vi "winFormsSubVI searchLayout.vi"(8 "error in (no error)":errorcluster, 11 "searchString":refnum<vi>) -> (0 "error out":errorcluster)   [LabVIEW 2018]
uses:
  PublicSubVI/Class/QMH/QMH.lvclass
panel:
  in  "cancelBtn":bool
  in  "searchBtn":bool
  in  "searchText":string caption="Search Text :"
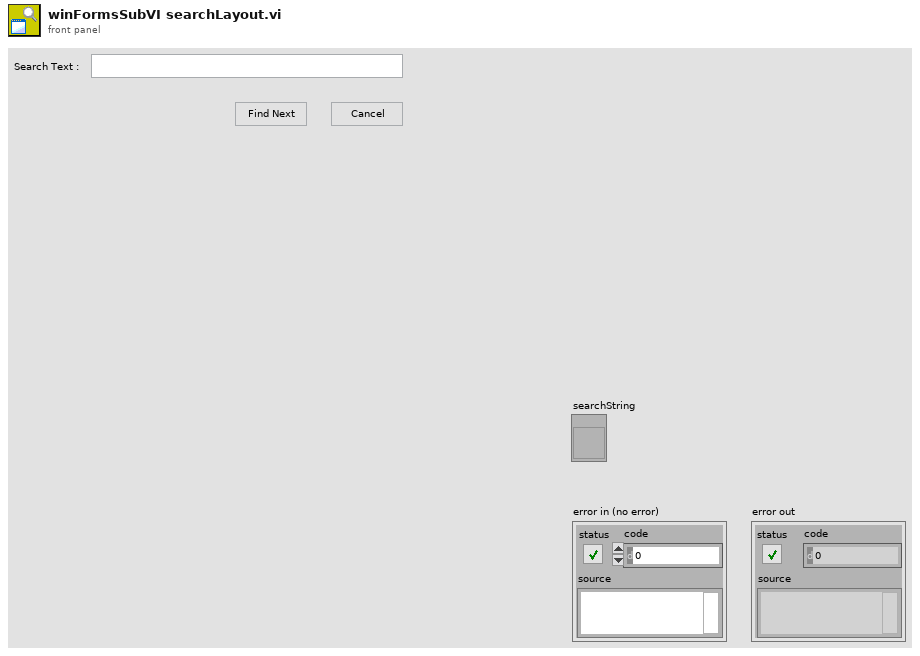
[diagram p1: front panel]
types:
  T1 = enum32{"Invalid", "Default", "Floating", "Floating/Auto-Hide", "Modal"}
  T2 = typedef "eventvkey.ctl" = enum16{"ASCII", "Enter", "Return", "Shift", "Ctrl", "Alt", "Cmd", "Opt", "Caps", "NumLock", "Clear", "Break", "Up", "Down", "Left", "Right", "Insert", "Delete", "Home", "End", "PageUp", "PageDown", "Escape", "Help", "Pause", "ScrollLock", "F1", "F2", "F3", "F4", "F5", "F6", "F7", "F8", "F9", "F10", "F11", "F12", "F13", "F14", "F15", "F16", "F17", "F18", "F19", "F20", "F21", "F22", "F23", "F24", "Play", "VolumeUp", "VolumeDown", "Mute", "Two Byte Char"}
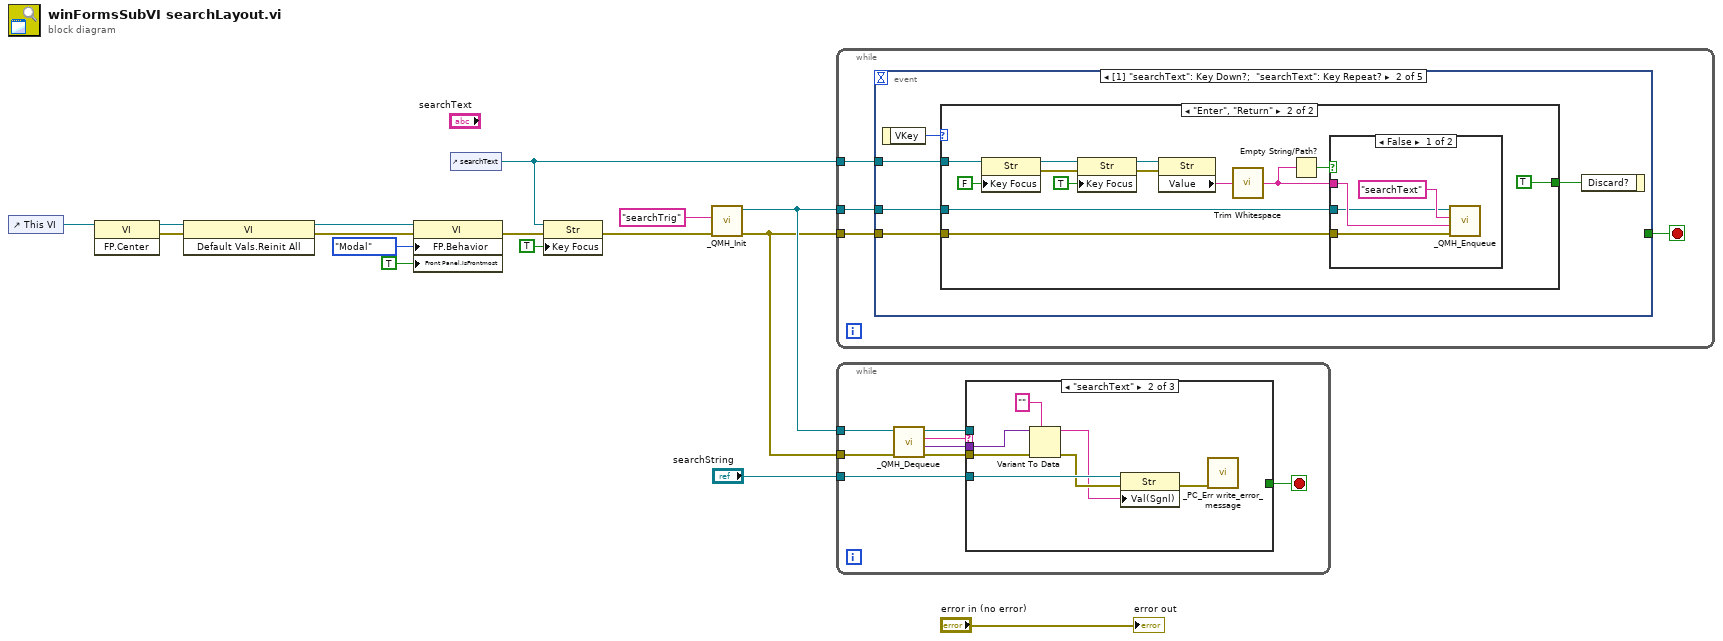
[diagram p0: block diagram]
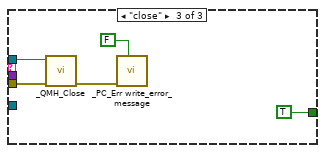
[diagram p3: hidden frame]
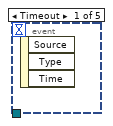
[diagram p4: hidden frame]
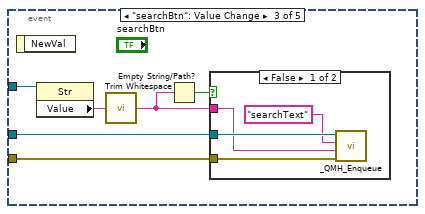
[diagram p7: hidden frame]
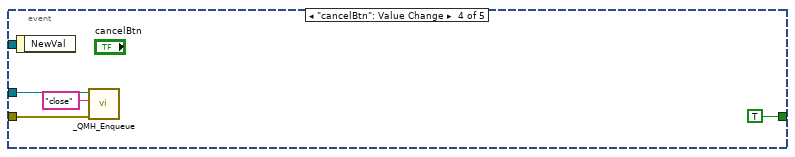
[diagram p9: hidden frame]
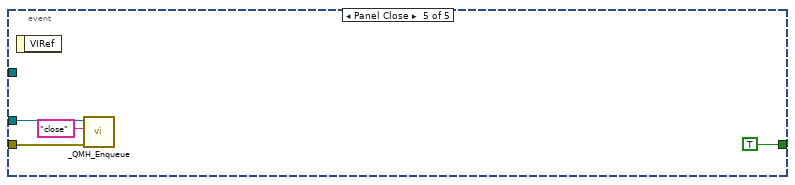
[diagram p10: hidden frame]
diagram:
  n1 = control-ref of="This VI"() -> (w9:refnum<vi>)
  n2 = invoke class="VI" method="FP.Center"(reference=w9) -> (reference out=w8:refnum<vi>, error out=w7:errorcluster)  [unwired: 2 in, 1 out]
  n3 = invoke class="VI" method="Default Vals.Reinit All"(reference=w8, error in=w7) -> (reference out=w5:refnum<vi>, error out=w6:errorcluster)  [unwired: 1 in, 1 out]
  n4 = property class="VI"(reference=w5, error in=w6, "FP.Behavior"=T1."Modal" ("Front Panel Window:Behavior"), "Front Panel.IsFrontmost"=TRUE ("Front Panel Window:Is Frontmost")) -> (error out=w2:errorcluster)  [unwired: 1 out]
  n5 = control-ref of="searchText"() -> (w4:refnum<vi>)
  n6 = property class="Str"(reference=w4, error in=w2, "Key Focus"=TRUE) -> (error out=w1:errorcluster)  [unwired: 1 out]
  n7 = call "_QMH_Init.vi"("error in (no error)"=w1, "name (unnamed)"="searchTrig") -> ("error out"=w14:errorcluster, "QMH out"=w15:refnum<class "QMH.lvclass">)  [unwired: 8 in]
  n8 = while {
    tunnel: w4 -> [w20]
    tunnel: w15 -> [w19]
    tunnel: w14 -> [w18]
    stop <- w17 stop-if-true
    n9 = event shown="[1] \"searchText\": Key Down?;  \"searchText\": Key Repeat?" {
      selector: _ -> [_ _ _ _ _]
      dyn-events: _ -> [_ _ _ _ _]
      timeout: _ -> [_ _ _ _ _]
      tunnel: w20 -> [_ w24 w46 _ _]
      tunnel: w19 -> [_ w23 w48 w56 w59]
      tunnel: w18 -> [_ w22 w47 w55 w58]
      tunnel: [_ _ _ TRUE TRUE] -> w17
      event Timeout {
        n10 = event-data() -> ()  [unwired: 1 in, 3 out]
      }
      event "searchText": Key Down?; "searchText": event type 3.0.x8000000b {
        n11 = event-data() -> ("VKey"=w25:T2)  [unwired: 1 in]
        n12 = case shown="\"Enter\", \"Return\"" w25 {
          tunnel: w24 -> [_ w31]
          tunnel: w23 -> [_ w36]
          tunnel: w22 -> [_ w35]
          tunnel: [_ TRUE] -> w21
          frame "ASCII", Default {
          }
          frame "Enter", "Return" {
            n13 = property class="Str"(reference=w31, "Key Focus"=FALSE) -> (reference out=w29:refnum<vi>, error out=w28:errorcluster)  [unwired: 1 in]
            n14 = property class="Str"(reference=w29, error in=w28, "Key Focus"=TRUE) -> (reference out=w27:refnum<vi>, error out=w26:errorcluster)
            n15 = property class="Str"(reference=w27, error in=w26) -> ("Value"=w37:string)  [unwired: 2 out]
            n16 = call <vilib>:"Trim Whitespace.vi"("string"=w37) -> ("trimmed string"=w34:string)  [unwired: 1 in]
            n17 = Empty String/Path?(string/path=w34) -> (empty?=w38:bool)
            n18 = case shown="False" w38 {
              tunnel: w34 -> [w41 _]
              tunnel: w36 -> [w40 _]
              tunnel: w35 -> [w39 _]
              frame False {
                n19 = call "_QMH_Enqueue.vi"("error in (no error)"=w39, "Data"=w41, "Msg"="searchText", "QMH in"=w40) -> ()  [unwired: 6 in, 2 out]
              }
              frame True {
              }
            }
          }
        }
        n20 = event-data("Discard?"=w21) -> ()  [unwired: 1 in, 1 out]
      }
      event "searchBtn": Value Change {
        n21 = event-data() -> ()  [unwired: 1 in, 1 out]
        n22 = property class="Str"(reference=w46) -> ("Value"=w45:string)  [unwired: 1 in, 2 out]
        n23 = call <vilib>:"Trim Whitespace.vi"("string"=w45) -> ("trimmed string"=w43:string)  [unwired: 1 in]
        n24 = Empty String/Path?(string/path=w43) -> (empty?=w44:bool)
        n25 = case shown="False" w44 {
          tunnel: w48 -> [w52 _]
          tunnel: w47 -> [w50 _]
          tunnel: w43 -> [w51 _]
          frame False {
            n26 = call "_QMH_Enqueue.vi"("error in (no error)"=w50, "Data"=w51, "Msg"="searchText", "QMH in"=w52) -> ()  [unwired: 6 in, 2 out]
          }
          frame True {
          }
        }
      }
      event "cancelBtn": Value Change {
        n27 = event-data() -> ()  [unwired: 1 in, 1 out]
        n28 = call "_QMH_Enqueue.vi"("error in (no error)"=w55, "Msg"="close", "QMH in"=w56) -> ()  [unwired: 7 in, 2 out]
      }
      event Panel Close {
        n29 = event-data() -> ()  [unwired: 1 in, 1 out]
        n30 = call "_QMH_Enqueue.vi"("error in (no error)"=w58, "Msg"="close", "QMH in"=w59) -> ()  [unwired: 7 in, 2 out]
      }
    }
  }
  n31 = while {
    tunnel: w15 -> [w68]
    tunnel: w14 -> [w67]
    tunnel: "searchString" -> [w61]
    stop <- w62 stop-if-true
    n32 = call "_QMH_Dequeue.vi"("error in (no error)"=w67, "QMH in"=w68) -> ("error out"=w63:errorcluster, "Data"=w65:variant, "Msg"=w66:string, "QMH out"=w64:refnum<class "QMH.lvclass">)  [unwired: 4 in, 2 out]
    n33 = case shown="\"searchText\"" w66 {
      tunnel: w65 -> [_ w74 _]
      tunnel: w64 -> [_ _ w80]
      tunnel: w63 -> [_ w73 w79]
      tunnel: [_ _ TRUE] -> w62
      tunnel: w61 -> [_ w75 _]
      frame Default {
      }
      frame "searchText" {
        n34 = Variant To Data(error in=w73, type="", Variant=w74) -> (data=w70:string, error out=w71:errorcluster)
        n35 = property class="Str"(reference=w75, error in=w71, "Val(Sgnl)"=w70) -> (error out=w69:errorcluster)  [unwired: 1 out]
        n36 = call "_PC_Err write_error_message.vi"("error in"=w69) -> ()  [unwired: 10 in, 1 out]
      }
      frame "close" {
        n37 = call "_QMH_Close.vi"("error in (no error)"=w79, "QMH in"=w80) -> ("error out"=w77:errorcluster)  [unwired: 9 in]
        n38 = call "_PC_Err write_error_message.vi"("show msg( T )"=FALSE, "error in"=w77) -> ()  [unwired: 9 in, 1 out]
      }
    }
  }
  "error out" <- "error in (no error)"
